vi "Untitled 1 (SubVI).vi"(10 "Value":dbl format="%#_13g", 11 "Slide in":refnum<vi>) -> ()   [LabVIEW 2014]
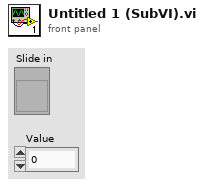
[diagram p1: front panel]
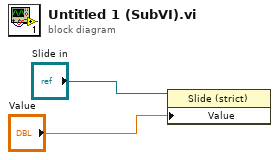
[diagram p0: block diagram]
diagram:
  n1 = property class="Slide (strict)"(reference="Slide in", "Value"="Value") -> ()  [unwired: 1 in, 2 out]
